vi "Route_mapping_global.vi"() -> ()   [LabVIEW 2013]
uses:
  Exclude_cluster.ctl
  Box_size.ctl
  Exclusion_type.ctl
  Route_Display_Mode.ctl
panel:
  in  "Traverse Setup":string
  in  "Probe Support":T1=[{"Max"=15001.0, "Min"=12000.0}, {"Max"=1000.0, "Min"=-1000.0}, {"Max"=700.0, "Min"=0.0}] {"Min" format="%#.1f"; "Max" format="%#.1f"}
  in  "Display Mode":T2=enum."Display View on Crash"
  in  "Entire Space":T1=[{"Max"=15001.0, "Min"=12000.0}, {"Max"=1000.0, "Min"=-1000.0}, {"Max"=700.0, "Min"=0.0}] {"Min" format="%#.1f"; "Max" format="%#.1f"}
  in  "Probe Volume":T1=[{"Max"=15.0, "Min"=-15.0}, {"Max"=250.0, "Min"=0.0}, {"Max"=15.0, "Min"=-15.0}] {"Min" format="%#.1f"; "Max" format="%#.1f"}
  in  "Exclude Array":T3[](array[typedef]) {"Sizes"."Min" format="%#.1f"; "Sizes"."Max" format="%#.1f"}
  # "(Relative to measurement position)"
  # "X                           Y                          Z"
  # "X                           Y                          Z"
  # "X                           Y                          Z"
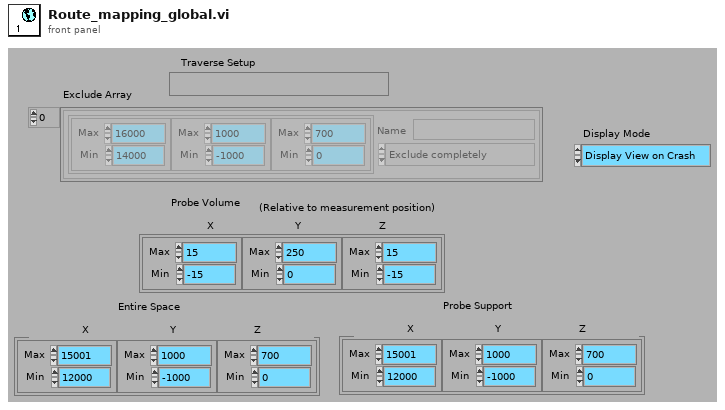
[diagram p1: front panel]
types:
  T1 = typedef "Box_size.ctl" = cluster{"Max":dbl, "Min":dbl}[]
  T2 = typedef "Route_Display_Mode.ctl" = enum16{"Display View Always", "Display View on Crash"}
  T3 = typedef "Exclude_cluster.ctl" = cluster{"Sizes":T1, "Name":string, "Exclude Type":T4}
  T4 = typedef "Exclusion_type.ctl" = enum16{"Exclude completely", "Allow only vertical moves"}
diagram:
